vi "set_Ic_sim_parameter (gyue@illinois.edu).vi"(8 "error in (no error)":errorcluster, 11 "Parameters":T1 {"temperature K" step=0.01}) -> (0 "error out":errorcluster)   [LabVIEW 2020]
uses:
  paramaters2.ctl
  ygDLL.dll
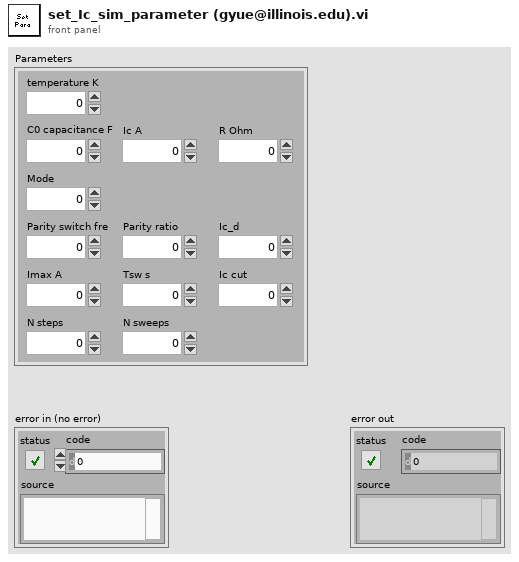
[diagram p1: front panel]
types:
  T1 = typedef "paramaters2.ctl" = cluster{"temperature K":dbl, "C0 capacitance F":dbl, "Ic A":dbl, "R Ohm":dbl, "Mode":i32, "Parity switch fre":dbl, "Parity ratio":dbl, "Imax A":dbl, "Tsw s":dbl, "N steps":i32, "Ic_d":dbl, "N sweeps":i32, "Ic cut":dbl}
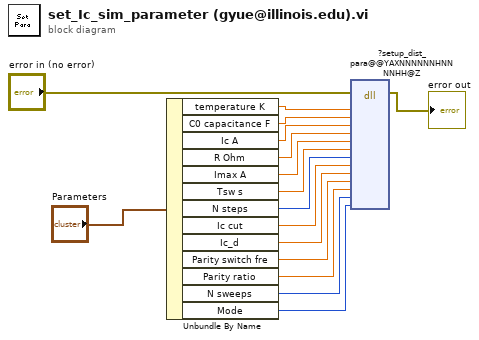
[diagram p0: block diagram]
diagram:
  n1 = Unbundle By Name("Parameters") -> ("temperature K"=w3:dbl, "C0 capacitance F"=w4:dbl, "Ic A"=w5:dbl, "R Ohm"=w6:dbl, "Imax A"=w7:dbl, "Tsw s"=w8:dbl, "N steps"=w9:i32, "Ic cut"=w10:dbl, "Ic_d"=w11:dbl, "Parity switch fre"=w12:dbl, "Parity ratio"=w13:dbl, "N sweeps"=w14:i32, "Mode"=w15:i32)
  n2 = dll-call lib="C:/Users/gyue/Box/Guang Yue uiuc research box folder/computation/Labview simulation GUI/ygDLL.dll" fn="?setup_dist_para@@YAXNNNNNNHNNNNHH@Z"(error in="error in (no error)", "temp"=w3, "c"=w4, "ic"=w5, "r"=w6, "im"=w7, "tsw"=w8, "nstep"=w9, "lcut"=w10, "ic_d"=w11, "fparity"=w12, "icr"=w13, "sweeps"=w14, "mode"=w15) -> (error out=→"error out":errorcluster)  [unwired: 16 in, 1 out]
